vi "MessageName.vi"() -> (2 "MessageName":string)   [LabVIEW 2020, in "TwoDoubles.lvlib"]
uses:
  TwoDoubles.lvlib
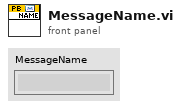
[diagram p1: front panel]
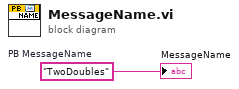
[diagram p0: block diagram]
diagram:
  w1 = "TwoDoubles"  # PB MessageName
  "MessageName" <- w1
